vi "Start Module.vi"(8 "error in (no error)":errorcluster) -> (0 "error out":errorcluster, 3 "isModuleRunning?":bool)   [LabVIEW 2014, in "Chart Module.lvlib"]
uses:
  Chart Module.lvlib
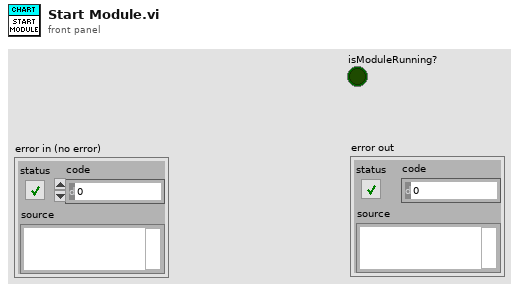
[diagram p1: front panel]
types:
  T1 = enum32{"Bad", "Idle", "Run top level", "Running"}
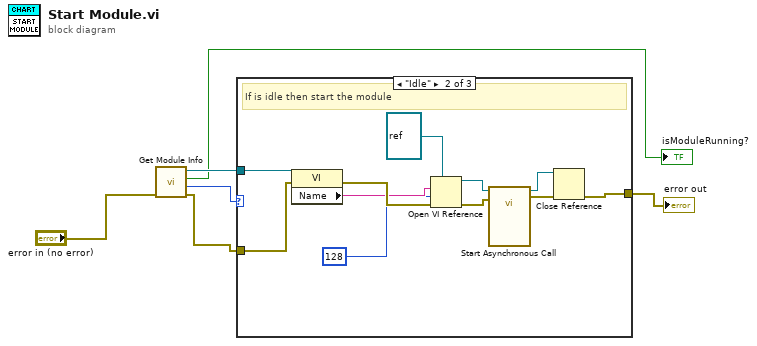
[diagram p0: block diagram]
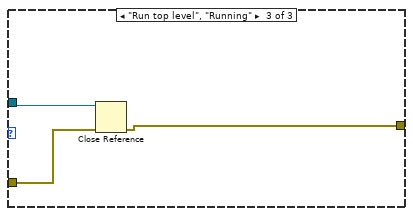
[diagram p3: hidden frame]
diagram:
  n1 = call "Get Module Info.vi"("error in (no error)"="error in (no error)") -> ("error out"=w4:errorcluster, "Execution State"=w6:T1, "isModuleRunning?"=→"isModuleRunning?":bool, "Module Ref"=w5:refnum<vi>)  [unwired: 7 in]
  n2 = case shown="\"Idle\"" w6 {
    tunnel: w5 -> [_ w16 w21]
    tunnel: w4 -> [w7 w9 w20]
    tunnel: [w7 w18 w19] -> w3
    frame "Bad", Default {
      # "Pending create constant error"
    }
    frame "Idle" {
      # "If is idle then start the module"
      n3 = property class="VI"(reference=w16, error in=w9) -> (error out=w15:errorcluster, "Name"=w10:string)  [unwired: 1 out]
      n4 = Open VI Reference(type specifier VI Refnum (for type only)=refnum<vi> refnum, vi path=w10, options=128, error in (no error)=w15) -> (vi reference=w14:refnum<vi>, error out=w11:errorcluster)  [unwired: 2 in]
      n5 = call-by-ref "Start Asynchronous Call"(reference=w14, error in=w11) -> (reference out=w13:refnum<vi>, error out=w12:errorcluster)  [unwired: 12 in]
      n6 = Close Reference(reference=w13, error in (no error)=w12) -> (error out=w18:errorcluster)
    }
    frame "Run top level", "Running" {
      n7 = Close Reference(reference=w21, error in (no error)=w20) -> (error out=w19:errorcluster)
    }
  }
  "error out" <- w3
